vi "SiosIfmIsEdlenEnabled.vi"(1 "Channel":i32(knob) scale=0.0..10.0, 2 "Device Number":i32) -> (0 "Is Edlen Enabled":i32)   [LabVIEW 2009]
uses:
  siosifm.dll
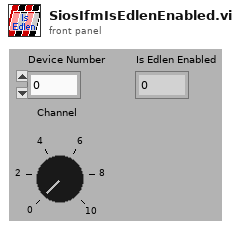
[diagram p1: front panel]
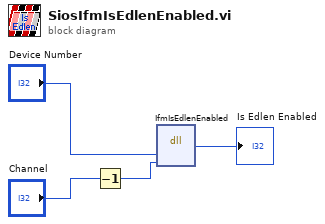
[diagram p0: block diagram]
diagram:
  n1 = Decrement(x="Channel") -> (x-1=w2:i32)
  n2 = dll-call lib="C:/WORK/Artem/RE-10/SIOS_IfmDLL/siosifm.dll" fn="IfmIsEdlenEnabled"("devNumber"="Device Number", "channel"=w2) -> ("IsEnabled"=→"Is Edlen Enabled":i32)  [unwired: 5 in, 2 out]
